vi "Check VNA Server.vi"(4 "error in (no error)":errorcluster) -> (0 "error out":errorcluster, 3 "Server On?":bool)   [LabVIEW 2023]
uses:
  <vilib>/Utility/error.llb/Trim Whitespace One-Sided.vi
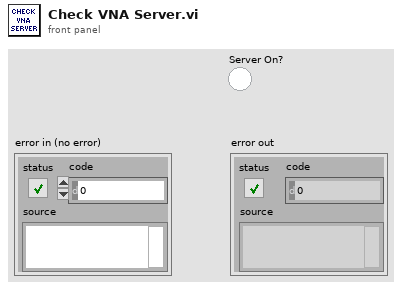
[diagram p1: front panel]
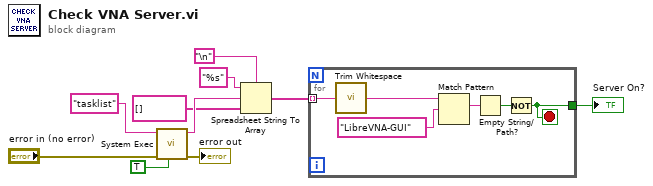
[diagram p0: block diagram]
diagram:
  n1 = call <vilib>:"System Exec.vi"("run minimized? (F)"=TRUE, "error in (no error)"="error in (no error)", "command line"="tasklist") -> ("error out"=→"error out":errorcluster, "standard output"=w8:string)  [unwired: 5 in, 2 out]
  n2 = Spreadsheet String To Array(delimiter (Tab)="\n", format string="%s", spreadsheet string=w8, array type (2D Dbl)=string[] []) -> (array=w4:string[])
  n3 = for {
    tunnel: w4 -> [w16] mode=indexing
    tunnel: [w11] -> w3
    stop <- w11 stop-if-true
    n4 = call <vilib>:"Trim Whitespace.vi"("string"=w16) -> ("trimmed string"=w15:string)  [unwired: 1 in]
    n5 = Match Pattern(string=w15, regular expression="LibreVNA-GUI") -> (match substring=w13:string)  [unwired: 1 in, 3 out]
    n6 = Empty String/Path?(string/path=w13) -> (empty?=w12:bool)
    n7 = Not(x=w12) -> (.not. x?=w11:bool)
  }
  "Server On?" <- w3
